vi "EXA_RF_Optimize_Range.vi"(8 "error in":errorcluster, 11 "VISA resource name":refnum<visa-resource-name>) -> (0 "error out":errorcluster, 3 "VISA resource name":refnum<visa-resource-name>)   [LabVIEW 2016]
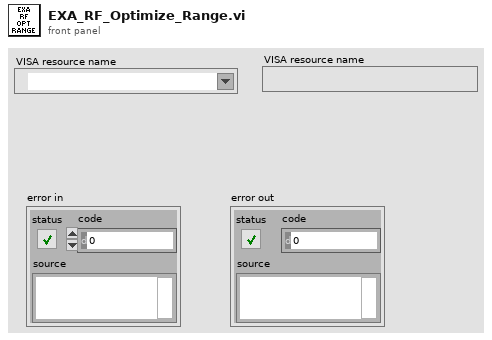
[diagram p1: front panel]
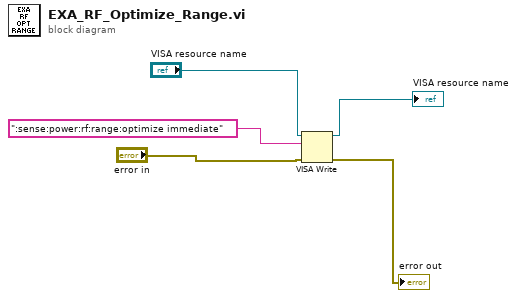
[diagram p0: block diagram]
diagram:
  n1 = VISA Write(VISA resource name="VISA resource name", write buffer=":sense:power:rf:range:optimize immediate" ("format string"), error in (no error)="error in") -> (VISA resource name out=→"VISA resource name":refnum<visa-resource-name>, error out=→"error out":errorcluster)  [unwired: 1 out]
